vi "test15.2-MappingRelationshipByLocalRegistration_WIthoutSubscriberName_State.vi"(8 "error in (no error)":errorcluster, 11 "TestCase in":refnum<class "testcase-CSMBroadcast.lvclass">) -> (0 "error out":errorcluster, 3 "TestCase out":refnum<class "testcase-CSMBroadcast.lvclass">)   [LabVIEW 2017, in "testcase-CSMBroadcast.lvclass"]
uses:
  testcase-CSMBroadcast.lvclass
  47fe1622-87c8-40c1-b9cf-9bbb5cd90bb5.vi
  <vilib>/addons/_JKI Toolkits/VI Tester/TestCase.llb/TestCase.lvclass
  src/user.lib/_NEVSTOP/Communicable State Machine(CSM)/Communicable State Machine.lvlib
  CSM/CSM-Testcase.lvlib
  C:/Program Files (x86)/National Instruments/LabVIEW 2017/vi.lib/addons/_JKI Toolkits/VI Tester/TestCase.llb/TestCase.lvclass
panel:
  out "Loop Count":i32
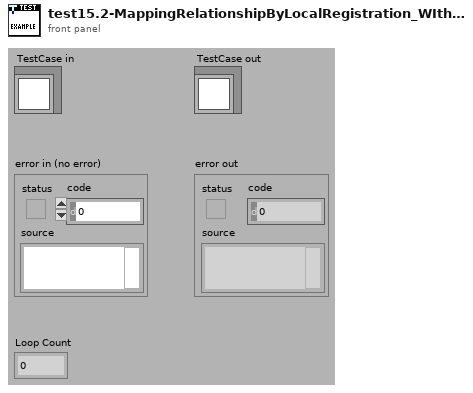
[diagram p1: front panel]
types:
  T1 = cluster{"Status":string, "Source CSM":string, "Target CSM":string, "Target API":string}[]
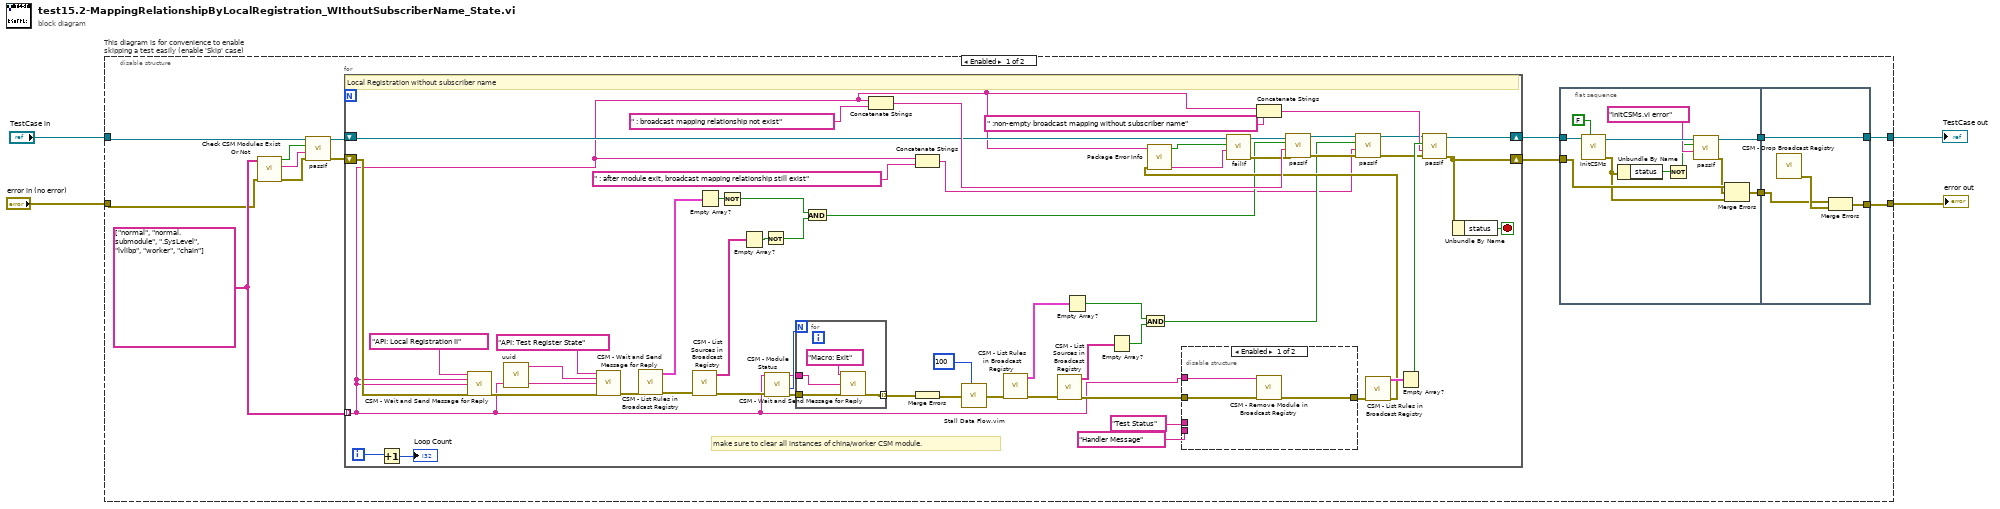
[diagram p0: block diagram]
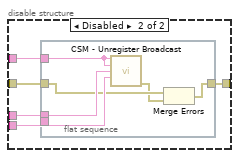
[diagram p2: hidden frame]
diagram:
  n1 = disable-structure "This diagram is for convenience to enable skipping a test easily (enable 'Skip' case)" shown="Enabled" {
    disable-tunnel: "TestCase in" -> [w14 w111]
    disable-tunnel: [w8 w109] -> w1
    disable-tunnel: [w7 w110] -> w3
    disable-tunnel: "error in (no error)" -> [w13 w108]
    frame Enabled {
      w15 = string[] ["normal", "normal.submodule", ".SysLevel", "lvlibp", "worker", "chain"]
      n2 = call "Check CSM Modules Exist Or Not.vi"("error in"=w13, "CSM names in"=w15) -> ("error out"=w16:errorcluster, "Debug string"=w17:string, "All Modules Exist?"=w18:bool)  [unwired: 7 in]
      n3 = call-dynamic "passIf.vi"("error in (no error)"=w16, "message (\"\")"=w17, "pass"=w18, "TestCase in"=w14) -> ("error out"=w5:errorcluster, "TestCase out"=w6:refnum<class "testcase-CSMBroadcast.lvclass">)  [unwired: 6 in]
      n4 = for {
        tunnel: w15 -> [w35] mode=indexing
        shift-right: [w70] -> w10
        shift-left: w6 -> [w50]
        shift-right: [w71] -> w9
        shift-left: w5 -> [w66]
        i -> [w80]
        stop <- w83 stop-if-true
        # "make sure to clear all instances of china/worker CSM module."
        # "Local Registration without subscriber name"
        n5 = Increment(x=w80) -> (x+1=→"Loop Count":i32)
        n6 = call "CSM - Wait and Send Message for Reply.vi"("State"="API: Local Registration II", "Arguments (\"\")"=w35, "Target Module"=w35, "Error In (No Error)"=w66) -> ("error out"=w88:errorcluster)  [unwired: 8 in, 3 out]
        n7 = call "uuid.vi"() -> ("UUID"=w86:string)  [unwired: 11 in]
        n8 = call "CSM - Wait and Send Message for Reply.vi"("State"="API: Test Register State", "Arguments (\"\")"=w86, "Target Module"=w35, "Error In (No Error)"=w88) -> ("error out"=w85:errorcluster)  [unwired: 8 in, 3 out]
        n9 = call "CSM - List Rules in Broadcast Registry.vi"("error in (no error)"=w85) -> ("error out"=w82:errorcluster, "Rule Entries"=w78:T1)  [unwired: 8 in, 1 out]
        n10 = call "CSM - List Sources in Broadcast Registry.vi"("error in (no error)"=w82) -> ("error out"=w63:errorcluster, "Broadcast Names"=w75:string[])  [unwired: 9 in]
        n11 = Empty Array?(array=w78) -> (empty?=w77:bool)
        n12 = Not(x=w77) -> (.not. x?=w48:bool)
        n13 = Empty Array?(array=w75) -> (empty?=w76:bool)
        n14 = Not(x=w76) -> (.not. x?=w47:bool)
        n15 = call "CSM - Module Status.vi"("Error In"=w63, "CSM Name"=w35) -> ("error out"=w62:errorcluster, "#Nodes"=w65:i32, "CSM Name (Dup)"=w64:string)  [unwired: 5 in, 2 out]
        n16 = for {
          N: w65 -> [_]
          tunnel: [w92] -> w84 mode=indexing
          tunnel: w64 -> [w91]
          tunnel: w62 -> [w90]
          n17 = call "CSM - Wait and Send Message for Reply.vi"("State"="Macro: Exit", "Target Module"=w91, "Error In (No Error)"=w90) -> ("error out"=w92:errorcluster)  [unwired: 9 in, 3 out]
        }
        n18 = And(x=w48, y=w47) -> (x .and. y?=w46:bool)
        n19 = Concatenate Strings(w35, " : broadcast mapping relationship not exist" ("string")) -> (w58:string)
        n20 = Concatenate Strings(w35, " : after module exit, broadcast mapping relationship still exist" ("string")) -> (w34:string)
        n21 = Merge Errors(w84) -> (w57:errorcluster)
        n22 = call "Stall Data Flow.vim"("value in"=w57, "milliseconds to wait"=u32 100) -> ("value out"=w56:errorcluster)  [unwired: 1 out]
        n23 = call "CSM - List Rules in Broadcast Registry.vi"("error in (no error)"=w56) -> ("error out"=w81:errorcluster, "Rule Entries"=w41:T1)  [unwired: 8 in, 1 out]
        n24 = call "CSM - List Sources in Broadcast Registry.vi"("error in (no error)"=w81) -> ("error out"=w74:errorcluster, "Broadcast Names"=w40:string[])  [unwired: 9 in]
        n25 = Empty Array?(array=w41) -> (empty?=w39:bool)
        n26 = Empty Array?(array=w40) -> (empty?=w38:bool)
        n27 = And(x=w39, y=w38) -> (x .and. y?=w37:bool)
        n28 = disable-structure shown="Enabled" {
          disable-tunnel: w74 -> [w96 w98]
          disable-tunnel: [w95 w97] -> w69
          disable-tunnel: w35 -> [w94 w99]
          disable-tunnel: "Test Status" ("Status") -> [_ w101]
          disable-tunnel: "Handler Message" ("Response Message (If \"\", Same as Source Message)") -> [_ w100]
          frame Enabled {
            n29 = call "CSM - Remove Module in Broadcast Registry.vi"("CSM Name"=w94, "Error In"=w96) -> ("error out"=w95:errorcluster)  [unwired: 12 in, 1 out]
          }
          frame Disabled {
            n30 = flat-sequence {
              tunnel: w101 -> [w107]
              tunnel: w100 -> [w106]
              tunnel: w99 -> [w105]
              tunnel: w98 -> [w104]
              tunnel: [w102] -> w97
              frame #0 {
                n31 = call "CSM - Unregister Broadcast.vi"("CSM Name(Empty for Broadcast Event)"=w105, "Source CSM Name (* as Default)"=w105, "Trigger"=w107, "API (\"*\" as Default)"=w106) -> ("error out"=w103:errorcluster)  [unwired: 10 in, 1 out]
                n32 = Merge Errors(w104, w103) -> (w102:errorcluster)
              }
            }
          }
        }
        n33 = Concatenate Strings(w35, " :non-empty broadcast mapping without subscriber name" ("string")) -> (w59:string)
        n34 = call "CSM - List Rules in Broadcast Registry.vi"("error in (no error)"=w69) -> ("error out"=w52:errorcluster, "Rule Entries"=w68:T1)  [unwired: 8 in, 1 out]
        n35 = call "Package Error Info.vi"("error in"=w52, "String in"=w35) -> ("packed error info out"=w54:string, "error status"=w53:bool)  [unwired: 8 in]
        n36 = call-dynamic "failIf.vi"("message (\"\")"=w54, "fail"=w53, "TestCase in"=w50) -> ("error out"=w51:errorcluster, "TestCase out"=w49:refnum<class "testcase-CSMBroadcast.lvclass">)  [unwired: 7 in]
        n37 = call-dynamic "passIf.vi"("error in (no error)"=w51, "message (\"\")"=w58, "pass"=w46, "TestCase in"=w49) -> ("error out"=w43:errorcluster, "TestCase out"=w45:refnum<class "testcase-CSMBroadcast.lvclass">)  [unwired: 6 in]
        n38 = call-dynamic "passIf.vi"("error in (no error)"=w43, "message (\"\")"=w34, "pass"=w37, "TestCase in"=w45) -> ("error out"=w42:errorcluster, "TestCase out"=w44:refnum<class "testcase-CSMBroadcast.lvclass">)  [unwired: 6 in]
        n39 = Empty Array?(array=w68) -> (empty?=w67:bool)
        n40 = call-dynamic "passIf.vi"("error in (no error)"=w42, "message (\"\")"=w59, "pass"=w67, "TestCase in"=w44) -> ("error out"=w71:errorcluster, "TestCase out"=w70:refnum<class "testcase-CSMBroadcast.lvclass">)  [unwired: 6 in]
        n41 = Unbundle By Name(w71) -> ("status"=w83:bool)
      }
      n42 = flat-sequence {
        tunnel: w10 -> [w29]
        tunnel: [w26] -> w12
        tunnel: w9 -> [w23]
        tunnel: [w20] -> w11
        tunnel: w12 -> [w32]
        tunnel: [w32] -> w8
        tunnel: [w31] -> w7
        tunnel: w11 -> [w30]
        frame #0 {
          n43 = call "InitCSMs.vi"("Enable building lvlibp?"=FALSE, "testcase-CSMStatus in"=w29) -> ("error out"=w21:errorcluster, "testcase-CSMStatus out"=w27:refnum<class "testcase-CSMBroadcast.lvclass">)  [unwired: 8 in]
          n44 = Unbundle By Name(w21) -> ("status"=w25:bool)
          n45 = Not(x=w25) -> (.not. x?=w19:bool)
          n46 = call-dynamic "passIf.vi"("message (\"\")"="initCSMs.vi error" ("message (\"\")"), "pass"=w19, "TestCase in"=w27) -> ("error out"=w22:errorcluster, "TestCase out"=w26:refnum<class "testcase-CSMBroadcast.lvclass">)  [unwired: 7 in]
          n47 = Merge Errors(w23, w22, w21) -> (w20:errorcluster)
        }
        frame #1 {
          n48 = call "CSM - Drop Broadcast Registry.vi"() -> ("error out"=w33:errorcluster)  [unwired: 15 in]
          n49 = Merge Errors(w30, w33) -> (w31:errorcluster)
        }
      }
    }
    frame Disabled {
      # "skip test result while test is under development"
      n50 = call <vilib>:"skip.vi"("error in (no error)"=w108, "TestCase in"=w111) -> ("error out"=w110:errorcluster, "TestCase out"=w109:refnum<class "testcase-CSMBroadcast.lvclass">)  [unwired: 8 in]
    }
  }
  "error out" <- w3
  "TestCase out" <- w1
